vi "GetAcceleration.vi"(10 "sensors list":string[](array[string]), 11 "packet in":u8[](array[numeric])) -> (1 "accZ":i16, 2 "accY":i16, 3 "accX":i16)   [LabVIEW 2018]
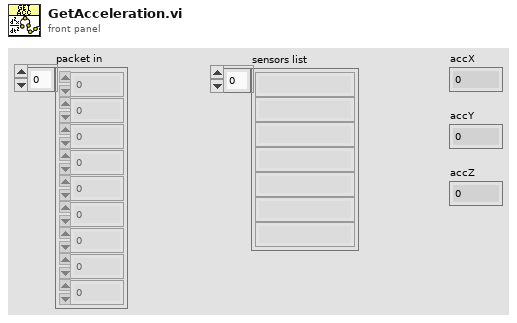
[diagram p1: front panel]
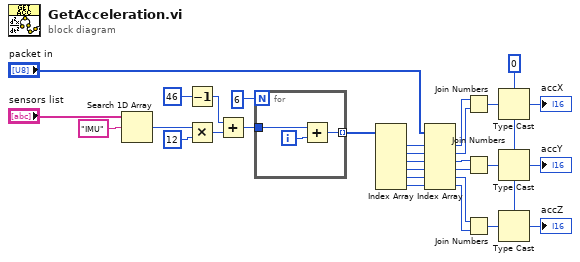
[diagram p0: block diagram]
diagram:
  w14 = i16 0 ("index")
  n1 = Search 1D Array(1D array="sensors list", element="IMU") -> (index of element=w17:i32)  [unwired: 1 in]
  n2 = Decrement(x=46) -> (x-1=w15:i32)
  n3 = Multiply(x=w17, y=12) -> (x*y=w16:i32)
  n4 = Add(x=w15, y=w16) -> (x+y=w22:i32)
  n5 = for {
    N: 6 -> [_]
    tunnel: w22 -> [w32]
    tunnel: [w31] -> w24 mode=indexing
    i -> [w33]
    n6 = Add(x=w32, y=w33) -> (x+y=w31:i32)
  }
  n7 = Index Array(array=w24) -> (element #1=w25:i32, element #2=w26:i32, element #3=w27:i32, element #4=w28:i32, element #5=w29:i32, element #6=w30:i32)  [unwired: 6 in]
  n8 = Index Array(array="packet in", index #1=w25, index #2=w26, index #3=w27, index #4=w28, index #5=w29, index #6=w30) -> (element #1=w12:u8, element #2=w11:u8, element #3=w10:u8, element #4=w9:u8, element #5=w8:u8, element #6=w7:u8)
  n9 = Join Numbers(hi=w12, lo=w11) -> ((hi.lo)=w3:u16)
  n10 = Join Numbers(hi=w10, lo=w9) -> ((hi.lo)=w2:u16)
  n11 = Join Numbers(hi=w8, lo=w7) -> ((hi.lo)=w1:u16)
  n12 = Type Cast(type=w14, x=w3) -> (*(type *) &x=→"accX":i16)
  n13 = Type Cast(type=w14, x=w2) -> (*(type *) &x=→"accY":i16)
  n14 = Type Cast(type=w14, x=w1) -> (*(type *) &x=→"accZ":i16)
